vi "编译图形.vi"(8 "error in (no error)":errorcluster caption="错误输入（无错误）", 11 "程序 输入":refnum<class "程序.lvclass">) -> (0 "error out":errorcluster caption="错误输出", 3 "程序 输出":refnum<class "程序.lvclass">)   [LabVIEW 2020, in "程序.lvclass"]
uses:
  D:/SuperPython-master/ScintillaNET.dll
  ScintillaNET.dll
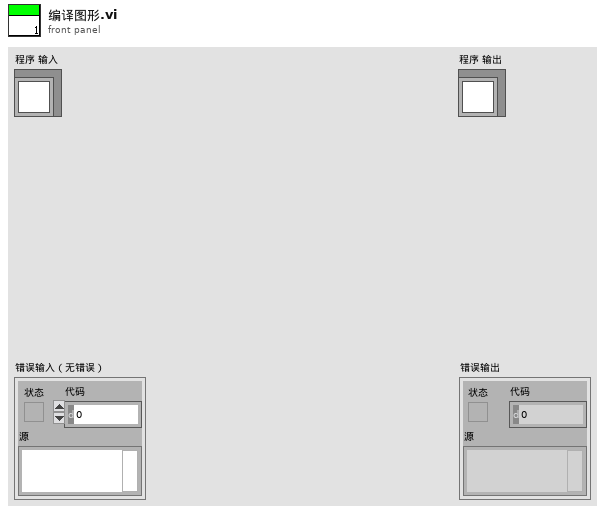
[diagram p1: front panel]
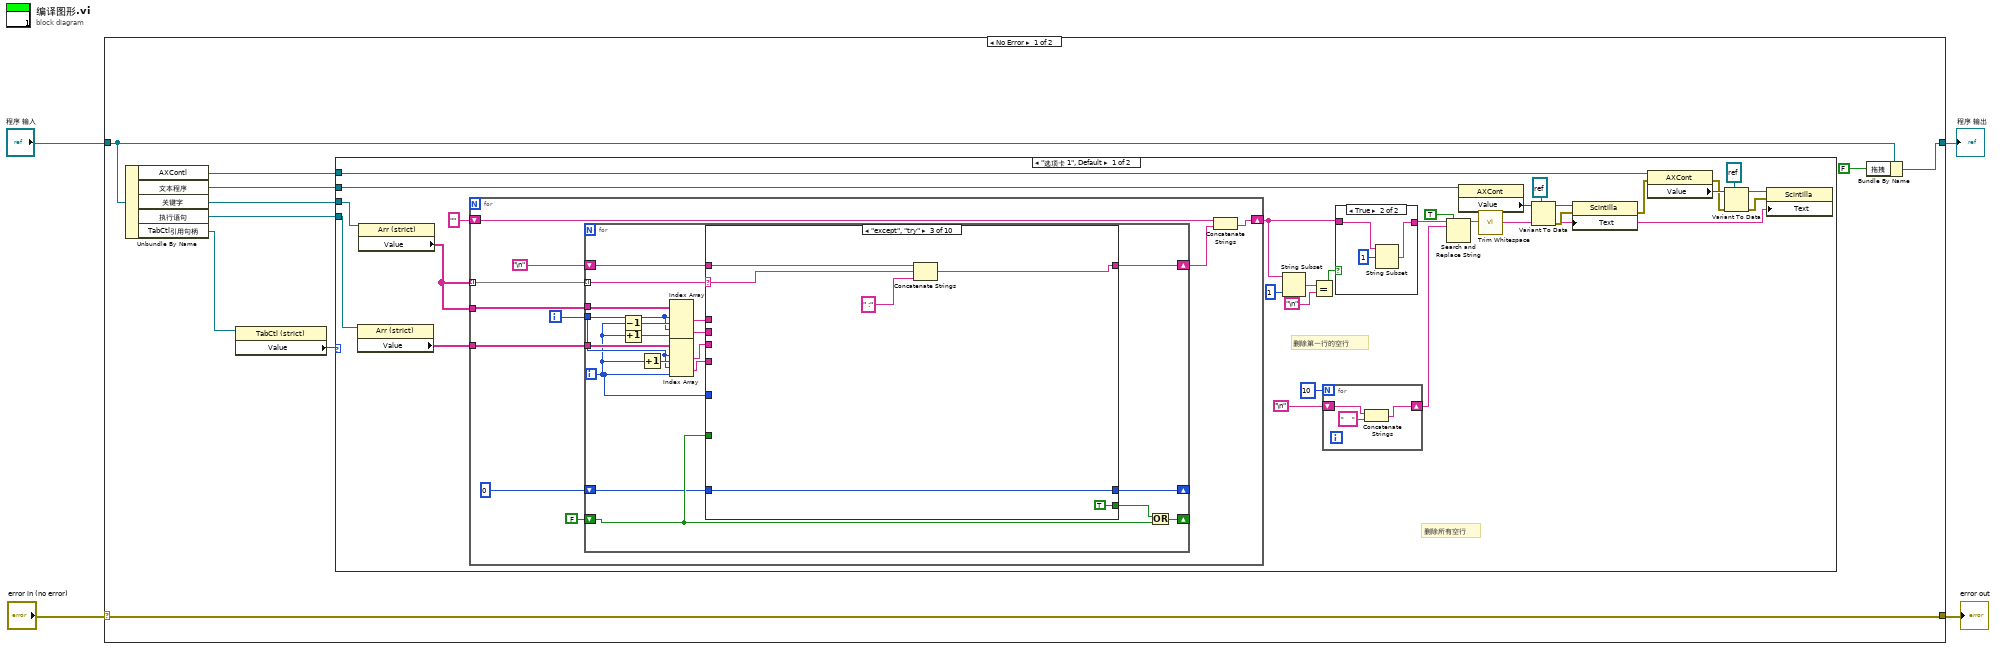
[diagram p0: block diagram]
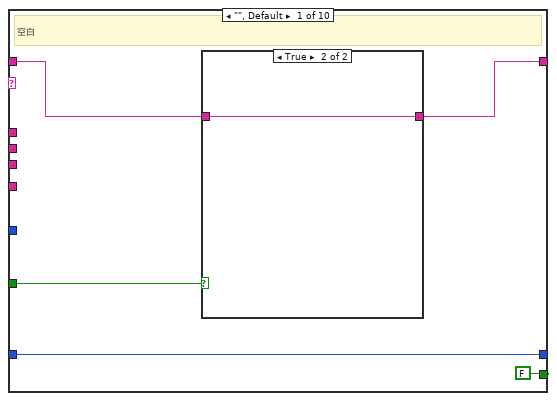
[diagram p3: hidden frame]
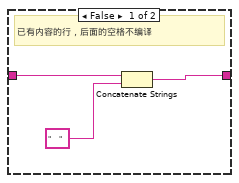
[diagram p4: hidden frame]
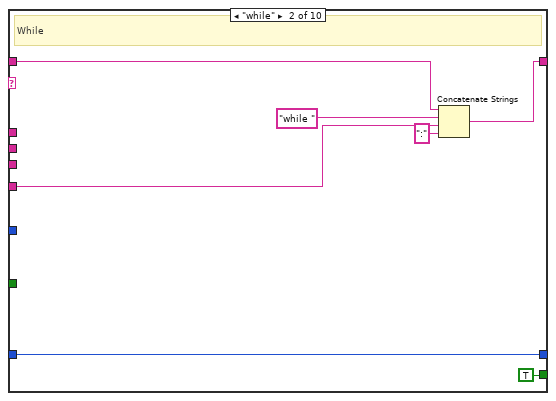
[diagram p5: hidden frame]
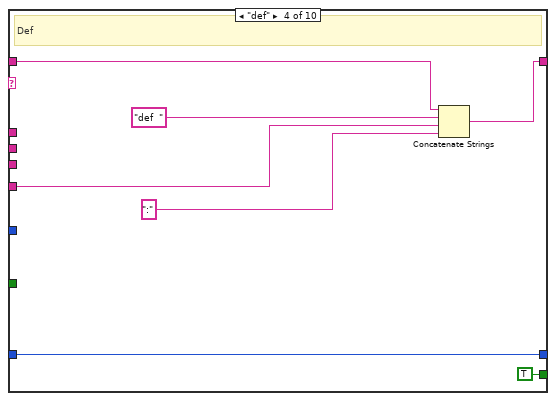
[diagram p6: hidden frame]
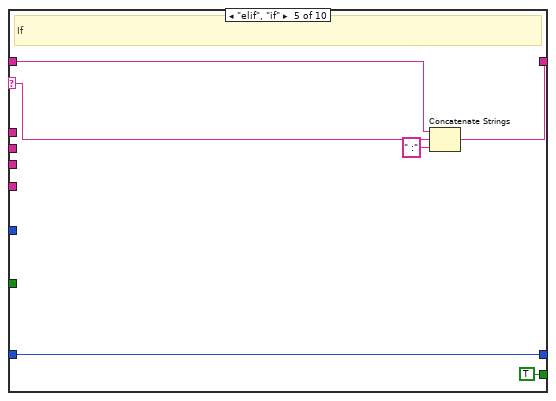
[diagram p7: hidden frame]
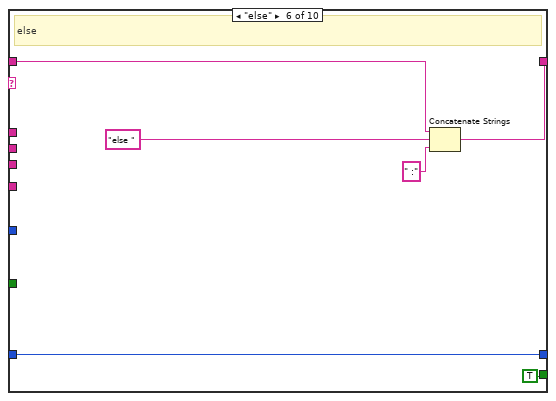
[diagram p8: hidden frame]
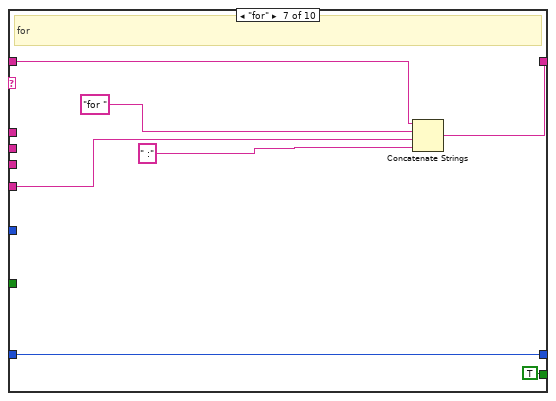
[diagram p9: hidden frame]
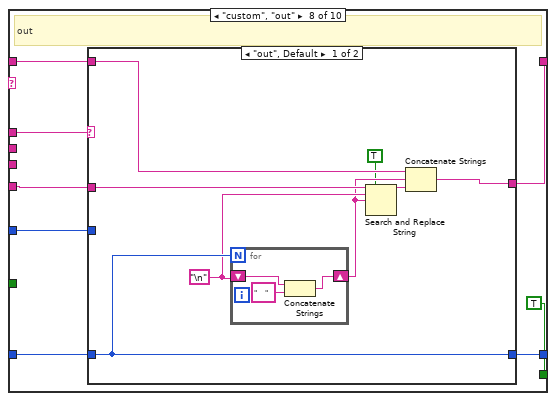
[diagram p10: hidden frame]
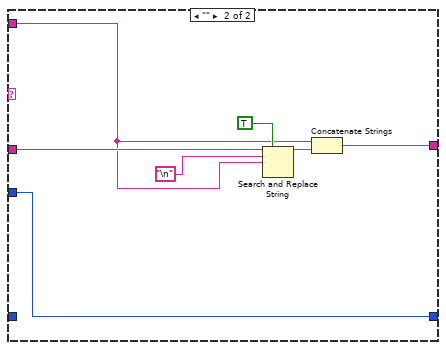
[diagram p11: hidden frame]
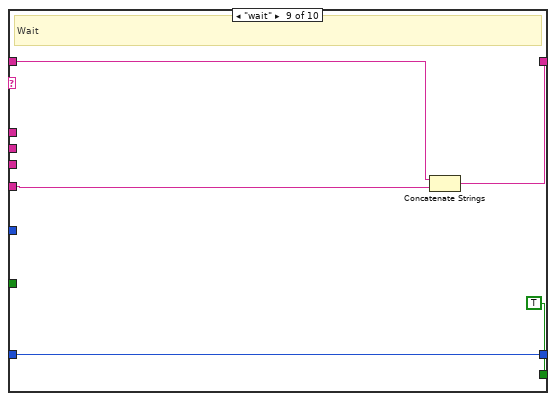
[diagram p12: hidden frame]
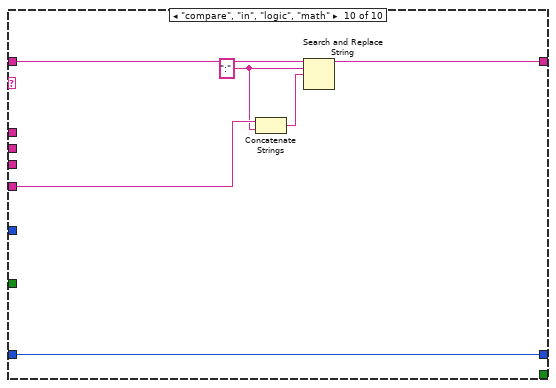
[diagram p13: hidden frame]
diagram:
  n1 = case shown="No Error" "error in (no error)" {
    selector: "error in (no error)" -> [w14 w166]
    tunnel: [w14 w166] -> w3
    tunnel: [w8 w165] -> w1
    tunnel: "程序 输入" -> [w10 w165]
    frame No Error {
      n2 = Unbundle By Name(w10) -> ("AXContl"=w7:refnum<vi>, "文本程序"=w11:refnum<vi>, "关键字"=w13:refnum<vi>, "执行语句"=w12:refnum<vi>, "TabCtl引用句柄"=w5:refnum<vi>)
      n3 = property class="TabCtl (strict)"(reference=w5) -> ("Value"=w6:enum32{"选项卡 1", "选项卡 2"})  [unwired: 1 in, 2 out]
      n4 = case shown="\"选项卡 1\", Default" w6 {
        tunnel: w13 -> [w40 _]
        tunnel: w12 -> [w39 _]
        tunnel: w11 -> [w38 _]
        tunnel: w7 -> [w24 _]
        frame "选项卡 1", Default {
          # "删除所有空行"
          # "删除第一行的空行"
          n5 = property class="Arr (strict)"(reference=w39) -> ("Value"=w41:string[][])  [unwired: 1 in, 2 out]
          n6 = property class="Arr (strict)"(reference=w40) -> ("Value"=w42:string[][])  [unwired: 1 in, 2 out]
          n7 = for {
            tunnel: w42 -> [w60] mode=indexing
            tunnel: w41 -> [w59]
            shift-right: [w55] -> w34
            shift-left: "" -> [w56]
            tunnel: w42 -> [w58]
            i -> [w57]
            n8 = for {
              tunnel: w60 -> [w79] mode=indexing
              shift-right: [w75] -> w54
              shift-left: "\n" -> [w73]
              tunnel: w59 -> [w77]
              tunnel: w58 -> [w72]
              tunnel: w57 -> [w69]
              shift-right: [w65] -> _
              shift-left: FALSE -> [w63]
              shift-right: [w62] -> _
              shift-left: 0 -> [w61]
              i -> [w68]
              n9 = Decrement(x=w68) -> (x-1=w71:i32)
              n10 = Increment(x=w68) -> (x+1=w67:i32)
              n11 = Increment(x=w68) -> (x+1=w74:i32)
              n12 = Index Array(array=w72, index (row) #1=w69, index (col) #1=w71, index (row) #2=w69, index (col) #2=w67) -> (element #1=w70:string, element #2=w66:string)
              n13 = Index Array(array=w77, index (row) #1=w69, index (col) #1=w74, index (row) #2=w69, index (col) #2=w68) -> (element #1=w78:string, element #2=w76:string)
              n14 = case shown="\"except\", \"try\"" w79 {
                selector: w79 -> [_ _ w99 _ w110 _ _ _ _ _]
                tunnel: [w84 w93 w98 w106 w113 w117 w123 w133 w156 w159] -> w75
                tunnel: w78 -> [_ _ _ _ _ _ _ _ _ _]
                tunnel: w76 -> [_ w91 _ w105 _ _ w126 w135 w158 w162]
                tunnel: w73 -> [w83 w94 w100 w107 w114 w118 w124 w134 w157 w163]
                tunnel: w70 -> [_ _ _ _ _ _ _ w132 _ _]
                tunnel: w68 -> [_ _ _ _ _ _ _ w131 _ _]
                tunnel: w66 -> [_ _ _ _ _ _ _ _ _ _]
                tunnel: [FALSE TRUE TRUE TRUE TRUE TRUE TRUE TRUE TRUE _] -> w64
                tunnel: w63 -> [w81 _ _ _ _ _ _ _ _ _]
                tunnel: [w80 w89 w97 w102 w111 w115 w121 w129 w154 w164] -> w62
                tunnel: w61 -> [w80 w89 w97 w102 w111 w115 w121 w128 w154 w164]
                frame "", Default {
                  # "空白"
                  n15 = case shown="True" w81 {
                    tunnel: [w87 w88] -> w84
                    tunnel: w83 -> [w86 w88]
                    frame False {
                      # "已有内容的行，后面的空格不编译"
                      n16 = Concatenate Strings(w86, "    " ("字符串")) -> (w87:string)
                    }
                    frame True {
                    }
                  }
                }
                frame "while" {
                  # "While"
                  n17 = Concatenate Strings(w94, "while " ("字符串"), w91, ":" ("字符串")) -> (w93:string)
                }
                frame "except", "try" {
                  n18 = Concatenate Strings(w100, w99, " :" ("字符串")) -> (w98:string)
                }
                frame "def" {
                  # "Def"
                  n19 = Concatenate Strings(w107, "def  " ("字符串"), w105, ":" ("字符串")) -> (w106:string)
                }
                frame "elif", "if" {
                  # "If"
                  n20 = Concatenate Strings(w114, w110, " :" ("字符串")) -> (w113:string)
                }
                frame "else" {
                  # "else"
                  n21 = Concatenate Strings(w118, "else ", " :" ("字符串")) -> (w117:string)
                }
                frame "for" {
                  # "for"
                  n22 = Concatenate Strings(w124, "for " ("字符串"), w126, " :" ("字符串")) -> (w123:string)
                }
                frame "custom", "out" {
                  # "out"
                  n23 = case shown="\"out\", Default" w132 {
                    tunnel: w135 -> [w141 w149]
                    tunnel: w134 -> [w143 w147]
                    tunnel: [w142 w148] -> w133
                    tunnel: w131 -> [_ w153]
                    tunnel: [w140 w153] -> w129
                    tunnel: w128 -> [w140 _]
                    frame "out", Default {
                      w139 = "\n"
                      n24 = for {
                        N: w140 -> [_]
                        shift-right: [w145] -> w137
                        shift-left: w139 -> [w146]
                        n25 = Concatenate Strings(w146, "    " ("字符串")) -> (w145:string)
                      }
                      n26 = Search and Replace String(replace all?=TRUE ("替换全部？(F)"), input string=w141, search string=w139, replace string=w137) -> (result string=w138:string)  [unwired: 4 in, 3 out]
                      n27 = Concatenate Strings(w143, w137, w138) -> (w142:string)
                    }
                    frame "" {
                      n28 = Search and Replace String(replace all?=TRUE ("替换全部？(F)"), input string=w149, search string="\n", replace string=w147) -> (result string=w151:string)  [unwired: 4 in, 3 out]
                      n29 = Concatenate Strings(w147, w151) -> (w148:string)
                    }
                  }
                }
                frame "wait" {
                  # "Wait"
                  n30 = Concatenate Strings(w157, w158) -> (w156:string)
                }
                frame "compare", "in", "logic", "math" {
                  w161 = ":" ("搜索字符串")
                  n31 = Concatenate Strings(w162, w161) -> (w160:string)
                  n32 = Search and Replace String(input string=w163, search string=w161, replace string=w160) -> (result string=w159:string)  [unwired: 5 in, 3 out]
                }
              }
              n33 = Or(x=w64, y=w63) -> (x .or. y?=w65:bool)
            }
            n34 = Concatenate Strings(w56, w54) -> (w55:string)
          }
          n35 = String Subset(string=w34, length (rest)=1 ("长度（剩余）")) -> (substring=w36:string)  [unwired: 1 in]
          n36 = Equal?(x=w36, y="\n") -> (x = y?=w33:bool)
          n37 = for {
            N: 10 -> [_]
            shift-right: [w45] -> w29
            shift-left: "\n" -> [w46]
            n38 = Concatenate Strings(w46, "    " ("字符串")) -> (w45:string)
          }
          n39 = case shown="True" w33 {
            tunnel: w34 -> [w47 w50]
            tunnel: [w47 w48] -> w32
            frame False {
            }
            frame True {
              n40 = String Subset(string=w50, offset (0)=1 ("偏移量(0)")) -> (substring=w48:string)  [unwired: 1 in]
            }
          }
          n41 = Search and Replace String(replace all?=TRUE ("替换全部？(F)"), input string=w32, search string=w29) -> (result string=w27:string)  [unwired: 5 in, 3 out]
          n42 = property class="AXCont"(reference=w38) -> ("Value"=w19:variant)  [unwired: 1 in, 2 out]
          n43 = call <vilib>:"Trim Whitespace.vi"("string"=w27) -> ("trimmed string"=w18:string)  [unwired: 1 in]
          n44 = Variant To Data(type=refnum<k24> refnum ("文本编辑"), Variant=w19) -> (data=w20:refnum<k24>, error out=w21:errorcluster)  [unwired: 1 in]
          n45 = property class="Scintilla"(reference=w20, error in=w21, "Text"=w18) -> (error out=w17:errorcluster)  [unwired: 1 out]
          n46 = property class="AXCont"(reference=w24, error in=w17) -> (error out=w16:errorcluster, "Value"=w26:variant)  [unwired: 1 out]
          n47 = Variant To Data(error in=w16, type=refnum<k24> refnum ("Scintilla"), Variant=w26) -> (data=w23:refnum<k24>, error out=w15:errorcluster)
          n48 = property class="Scintilla"(reference=w23, error in=w15, "Text"=w18) -> ()  [unwired: 2 out]
        }
        frame "选项卡 2" {
        }
      }
      n49 = Bundle By Name(cluster=w10, "拖拽"=FALSE) -> (w8:refnum<class "程序.lvclass">)
    }
    frame Error {
    }
  }
  "error out" <- w3
  "程序 输出" <- w1
